vi "Add FIFO Publisher.vi"(7 "Channel Array in":refnum<class "CIFChannels.lvclass">[](array[class]), 8 "error in (no error)":errorcluster, 9 "New FIFO Instance Config":T2, 10 "Channel Name":string, 11 "CIFChannelMng in":refnum<class "CIFChannelMng.lvclass">) -> (0 "error out":errorcluster, 1 "Update OOB":bool=TRUE, 2 "FIFO Publisher":T1, 3 "CIFChannelMng out":refnum<class "CIFChannelMng.lvclass">, 5 "Channel Array out":refnum<class "CIFChannels.lvclass">[](array[class]))   [LabVIEW 2021, in "CIFChannelMng.lvclass"]
uses:
  CIFChannelMng.lvclass
  <vilib>/CIF Foundation/CIF Channels Core/CIFChannels/Typedef/Channel State.ctl
  <vilib>/CIF Foundation/CIF Channels Core/CIFChannels/CIFChannels.lvclass
  typedef/FIFO Publisher Return.ctl
  typedef/Errors Channel Manager.ctl
  <vilib>/CIF Foundation/CIF Channels Core/ChannelCommon/typedef/New FIFO Instance Configuration.ctl
  <vilib>/CIF Foundation/CIF Channels Core/ChannelCommon/ChannelCommon.lvlib
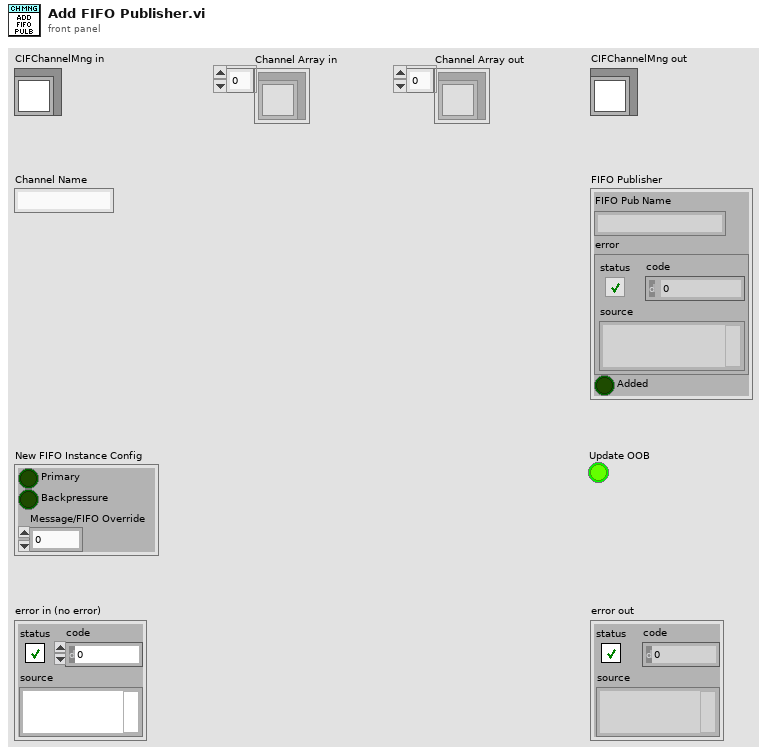
[diagram p1: front panel]
types:
  T1 = typedef "CIFChannelMng.lvclass/FIFO Publisher Return.ctl" = cluster{"FIFO Pub Name":string, "error":errorcluster, "Added":bool}
  T2 = typedef "ChannelCommon.lvlib/New FIFO Instance Configuration.ctl" = cluster{"Primary":bool, "Backpressure":bool, "Message/FIFO Override":u32}
  T3 = typedef "CIFChannelMng.lvclass/Errors Channel Manager.ctl" = enum16{"gRPC Server Not Found", "Duplicate Channel", "Missing Channel", "Incorrect Type", "Flatten Error", "Unflatten Data", "Channel Length", "Plugin Connection", "gRPC Server Connection", "FIFO Unflatten", "Required Override", "Remove Not Found", "Skipped due to warning", "Timeout FIFO Pub"}
  T4 = typedef "CIFChannels.lvclass/Channel State.ctl" = enum16{"Creating", "Disconnected", "Connecting", "Connected", "Destroyed"}
  T5 = typedef "CIFChannelMng.lvclass/Channel List for OOB.ctl" = cluster{"Name":string, "Direction":T6, "Type":string, "Connected?":bool, "Connected Name":string, "Custom Config Data":u8[], "Forced?":bool, "Pattern":T7}
  T6 = typedef "CIFChannels.lvclass/Direction.ctl" = enum16{"Publisher", "Subscriber"}
  T7 = typedef "ChannelCommon.lvlib/Channel Pattern.ctl" = enum16{"Unknown", "Tag", "FIFO", "MultiFIFO"}
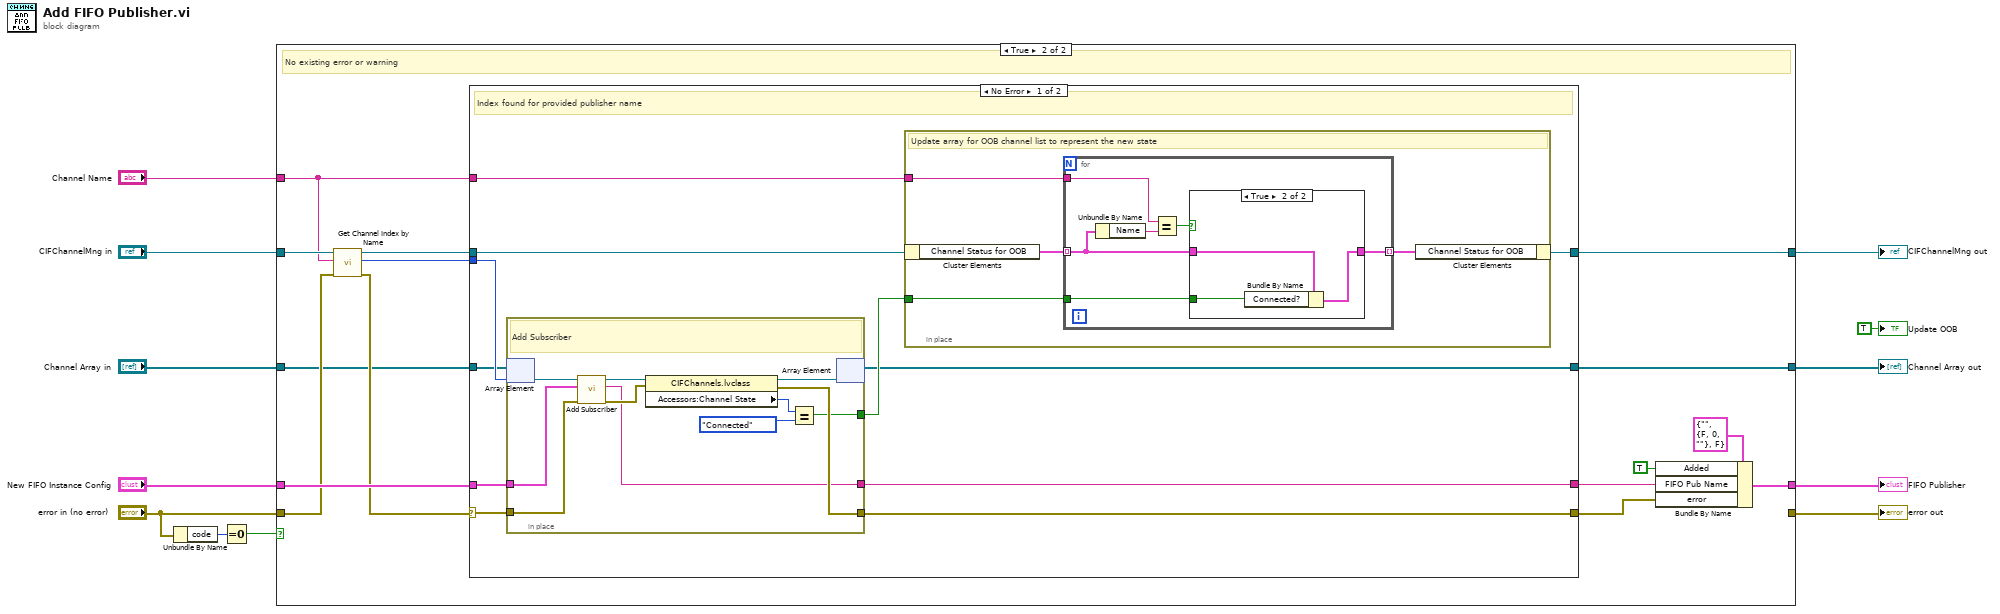
[diagram p0: block diagram]
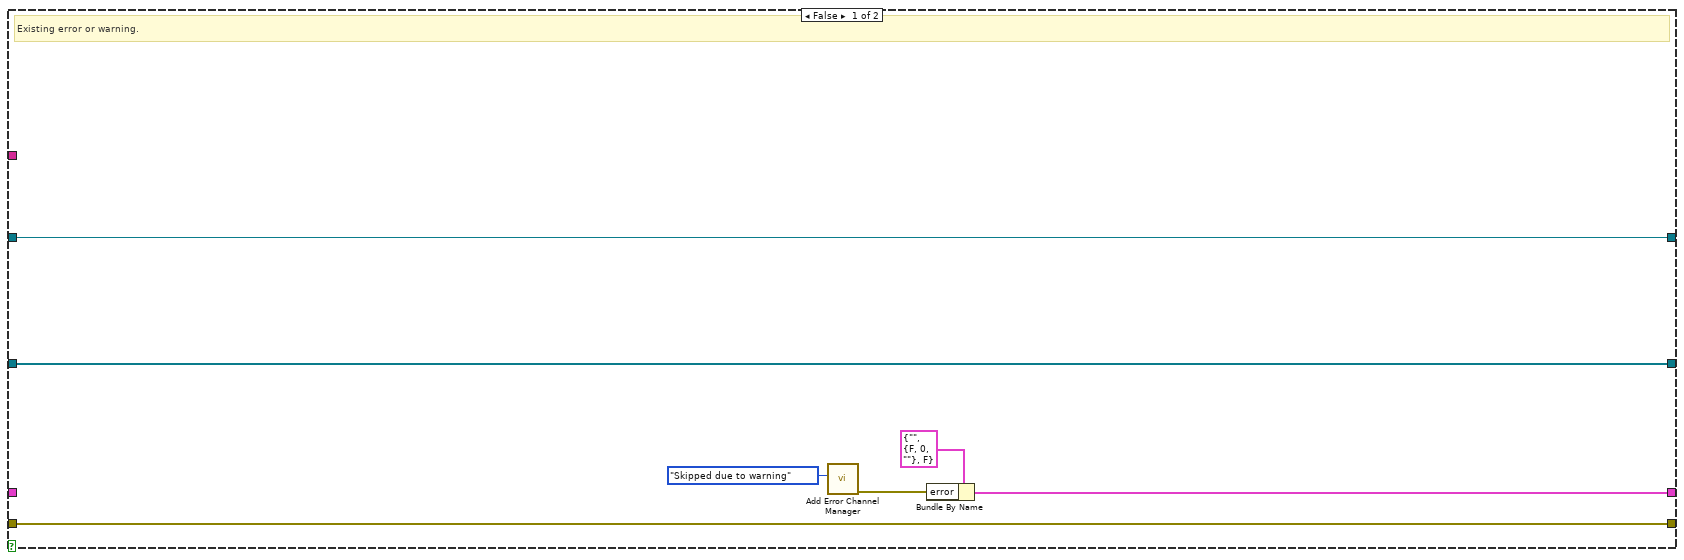
[diagram p2: hidden frame]
diagram:
  n1 = Unbundle By Name("error in (no error)") -> ("code"=w6:i32)
  n2 = Equal To 0?(x=w6) -> (x = 0?=w5:bool)
  n3 = case shown="True" w5 {
    tunnel: [w19 w30] -> w11
    tunnel: "CIFChannelMng in" -> [w19 w34]
    tunnel: "Channel Name" -> [_ w31]
    tunnel: [w18 _] -> w9
    tunnel: "New FIFO Instance Config" -> [_ w29]
    tunnel: [w16 w24] -> w7
    tunnel: "error in (no error)" -> [w18 w23]
    tunnel: "Channel Array in" -> [w13 w21]
    tunnel: [w13 w20] -> w1
    frame False {
      # "Existing error or warning."
      n4 = call "Add Error Channel Manager.vi"("Error"=Errors_Channel_Manager."Skipped due to warning") -> ("error out"=w15:errorcluster)  [unwired: 10 in]
      n5 = Bundle By Name(cluster=T1 {"FIFO Pub Name"="", "error"={"status"=FALSE, "code"=0, "source"=""}, "Added"=FALSE} ("New FIFO Publisher"), "error"=w15) -> (w16:T1)
    }
    frame True {
      # "No existing error or warning"
      n6 = call "Get Channel Index by Name.vi"("error in (no error)"=w23, "Channel Name"=w31, "CIFChannelMng in"=w34) -> ("error out"=w28:errorcluster, "Channel Index"=w32:i32, "CIFChannelMng out"=w33:refnum<class "CIFChannelMng.lvclass">)  [unwired: 6 in]
      n7 = case shown="No Error" w28 {
        selector: w28 -> [w40 w73]
        tunnel: w33 -> [w37 w72]
        tunnel: w32 -> [w45 _]
        tunnel: w31 -> [w44 _]
        tunnel: [w43 w72] -> w30
        tunnel: [w42 w73] -> w25
        tunnel: w29 -> [w41 _]
        tunnel: [w38 _] -> w26
        tunnel: w21 -> [w36 w71]
        tunnel: [w35 w71] -> w20
        frame No Error {
          # "Index found for provided publisher name"
          n8 = in-place {
            in-place-border: w40 -> [w54]
            in-place-border: [w50] -> w42
            in-place-border: w41 -> [w55]
            in-place-border: [w47] -> w39
            in-place-border: [w46] -> w38
            # "Add Subscriber"
            n9 = in-place-array #1(w36, w45) -> (w56:refnum<class "CIFChannels.lvclass">)
            n10 = call-dynamic "Add Subscriber.vi"("error in (no error)"=w54, "New FIFO Instance Config"=w55, "CIFChannels in"=w56) -> ("error out"=w51:errorcluster, "New Publisher"=w46:string, "CIFChannels out"=w53:refnum<class "CIFChannels.lvclass">)  [unwired: 6 in]
            n11 = property class="CIFChannels.lvclass"(reference=w53, error in=w51) -> (reference out=w52:refnum<class "CIFChannels.lvclass">, error out=w50:errorcluster, "Accessors:Channel State"=w48:T4)
            n12 = Equal?(x=w48, y=Channel_State."Connected" ("Channel State")) -> (x = y?=w47:bool)
            n13 = in-place-array #1(w52) -> (w35:refnum<class "CIFChannels.lvclass">[])  [unwired: 1 out]
          }
          n14 = in-place {
            in-place-border: w44 -> [w58]
            in-place-border: w39 -> [w57]
            # "Update array for OOB channel list to represent the new state"
            n15 = in-place-cluster #2(w37) -> ("Channel Status for OOB"=w60:T5[])
            n16 = for {
              tunnel: w60 -> [w65] mode=indexing
              tunnel: [w64] -> w59 mode=indexing
              tunnel: w58 -> [w63]
              tunnel: w57 -> [w61]
              n17 = Unbundle By Name(w65) -> ("Name"=w66:string)
              n18 = Equal?(x=w63, y=w66) -> (x = y?=w62:bool)
              n19 = case shown="True" w62 {
                tunnel: w65 -> [w67 w70]
                tunnel: [w67 w69] -> w64
                tunnel: w61 -> [_ w68]
                frame False {
                }
                frame True {
                  n20 = Bundle By Name(cluster=w70, "Connected?"=w68) -> (w69:T5)
                }
              }
            }
            n21 = in-place-cluster #2("Channel Status for OOB"=w59) -> (w43:refnum<class "CIFChannelMng.lvclass">)
          }
        }
        frame Error {
          # "Index by name created error"
        }
      }
      n22 = Bundle By Name(cluster=T1 {"FIFO Pub Name"="", "error"={"status"=FALSE, "code"=0, "source"=""}, "Added"=FALSE} ("New FIFO Publisher"), "Added"=TRUE, "FIFO Pub Name"=w26, "error"=w25) -> (w24:T1)
    }
  }
  "error out" <- w9
  "CIFChannelMng out" <- w11
  "FIFO Publisher" <- w7
  "Channel Array out" <- w1
  "Update OOB" <- TRUE ("Update OOB")
